vi "player1.vi"(11 "Char":i16) -> (3 "f":i32)   [LabVIEW 2014]
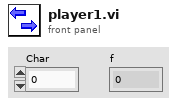
[diagram p1: front panel]
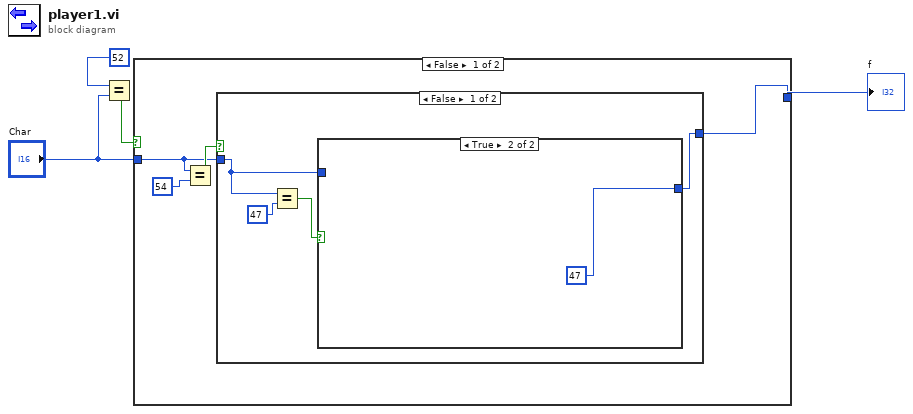
[diagram p0: block diagram]
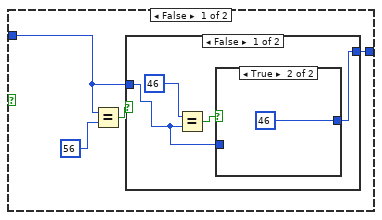
[diagram p2: hidden frame]
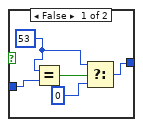
[diagram p3: hidden frame]
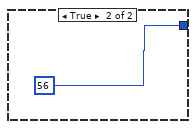
[diagram p4: hidden frame]
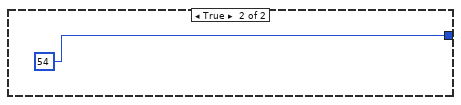
[diagram p5: hidden frame]
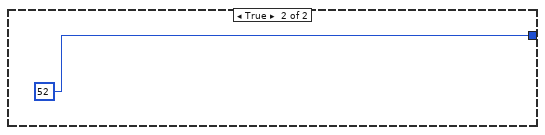
[diagram p6: hidden frame]
diagram:
  n1 = Equal?(x=52, y="Char") -> (x = y?=w2:bool)
  n2 = case shown="False" w2 {
    tunnel: "Char" -> [w5 _]
    tunnel: [w6 52] -> w4
    frame False {
      n3 = Equal?(x=w5, y=54) -> (x = y?=w7:bool)
      n4 = case shown="False" w7 {
        tunnel: [w10 54] -> w6
        tunnel: w5 -> [w9 _]
        frame False {
          n5 = Equal?(x=w9, y=47) -> (x = y?=w11:bool)
          n6 = case shown="True" w11 {
            tunnel: [w14 47] -> w10
            tunnel: w9 -> [w13 _]
            frame False {
              n7 = Equal?(x=w13, y=56) -> (x = y?=w15:bool)
              n8 = case shown="False" w15 {
                tunnel: [w18 56] -> w14
                tunnel: w13 -> [w19 _]
                frame False {
                  n9 = Equal?(x=46, y=w19) -> (x = y?=w17:bool)
                  n10 = case shown="True" w17 {
                    tunnel: [w22 46] -> w18
                    tunnel: w19 -> [w25 _]
                    frame False {
                      w23 = 53
                      n11 = Equal?(x=w23, y=w25) -> (x = y?=w24:bool)
                      n12 = Select(t=w23, s=w24, f=0) -> (s? t:f=w22:i32)
                    }
                    frame True {
                    }
                  }
                }
                frame True {
                }
              }
            }
            frame True {
            }
          }
        }
        frame True {
        }
      }
    }
    frame True {
    }
  }
  "f" <- w4
